vi "Read Core.vi"(8 "error in (no error)":errorcluster, 11 "Sequencer in":refnum<class "Sequencer.lvclass">) -> (0 "error out":errorcluster, 2 "Core":refnum<class "Sequencer Core.lvclass">, 3 "Sequencer out":refnum<class "Sequencer.lvclass">)   [LabVIEW 2020, in "Sequencer.lvlib" / "Sequencer.lvclass"]
doc: "Read the Sequencer Core from the Sequencer."
uses:
  Sequencer.lvclass
  Sequencer Core/Sequencer Core.lvclass
  Sequencer.lvclass/Sequencer.ctl
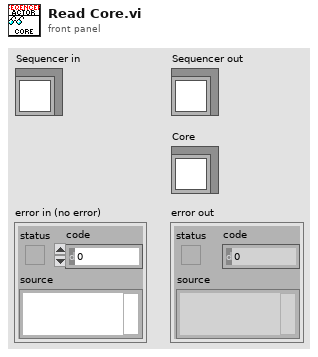
[diagram p1: front panel]
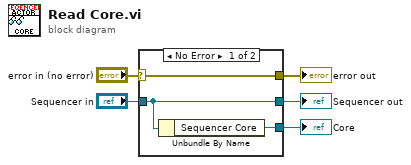
[diagram p0: block diagram]
diagram:
  n1 = case shown="No Error" "error in (no error)" {
    selector: "error in (no error)" -> [w8 w9]
    tunnel: [w8 w9] -> w4
    tunnel: [w7 w10] -> w2
    tunnel: "Sequencer in" -> [w7 w10]
    tunnel: [w6 _] -> w1
    frame No Error {
      n2 = Unbundle By Name(w7) -> ("Sequencer Core"=w6:refnum<class "Sequencer Core.lvclass">)
    }
    frame Error {
    }
  }
  "error out" <- w4
  "Sequencer out" <- w2
  "Core" <- w1
